vi "number1-state machine.vi"() -> ()   [LabVIEW 2014]
panel:
  out "Logined":bool
  in  "stop":bool
  out "array":bool[](array[boolean])
  in  "Button":T1
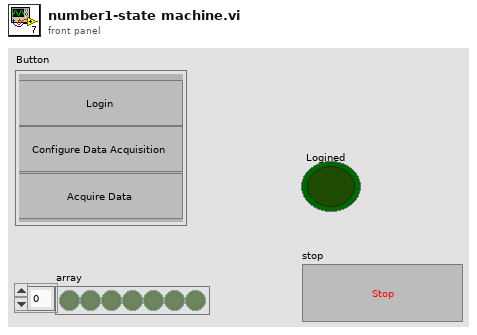
[diagram p1: front panel]
types:
  T1 = cluster{"OK Button":bool, "OK Button 2":bool, "OK Button 3":bool}
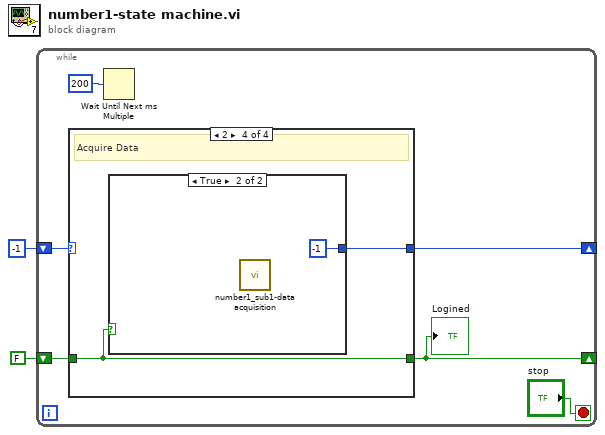
[diagram p0: block diagram]
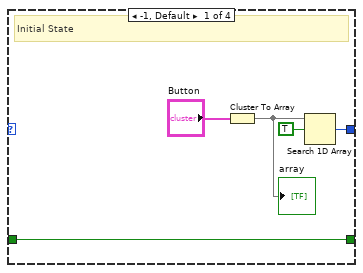
[diagram p2: hidden frame]
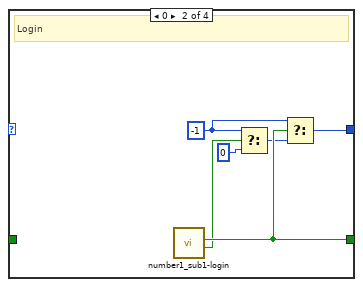
[diagram p3: hidden frame]
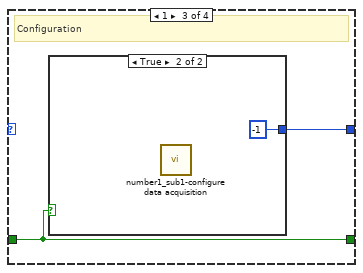
[diagram p4: hidden frame]
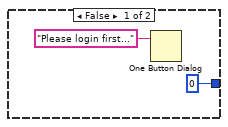
[diagram p5: hidden frame]
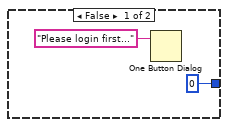
[diagram p6: hidden frame]
diagram:
  n1 = while {
    shift-right: [w7] -> _
    shift-left: -1 -> [w8]
    shift-right: [w6] -> _
    shift-left: FALSE -> [w5]
    stop <- "stop" stop-if-true
    n2 = case shown="2" w8 {
      tunnel: [w10 w18 w20 w25] -> w7
      tunnel: [w9 w19 w21 w26] -> w6
      tunnel: w5 -> [w9 _ w21 w26]
      frame -1, Default {
        # "Initial State"
        n3 = Cluster To Array(cluster="Button") -> (array=w12:bool[])
        "array" <- w12
        n4 = Search 1D Array(1D array=w12, element=TRUE) -> (index of element=w10:i32)  [unwired: 1 in]
      }
      frame 0 {
        w16 = -1
        # "Login"
        n5 = call "number1_sub1-login.vi"() -> ("UserCancelled"=w17:bool, "Correct"=w19:bool)  [unwired: 10 in]
        n6 = Select(t=w16, s=w17, f=0) -> (s? t:f=w14:i32)
        n7 = Select(t=w16, s=w19, f=w14) -> (s? t:f=w18:i32)
      }
      frame 1 {
        # "Configuration"
        n8 = case shown="True" w21 {
          tunnel: [0 -1] -> w20
          frame False {
            n9 = One Button Dialog(message="Please login first...") -> ()  [unwired: 1 in, 1 out]
          }
          frame True {
            n10 = call "number1_sub1-configure data acquisition.vi"() -> ()  [unwired: 8 in]
          }
        }
      }
      frame 2 {
        # "Acquire Data"
        n11 = case shown="True" w26 {
          tunnel: [0 -1 ("index of element")] -> w25
          frame False {
            n12 = One Button Dialog(message="Please login first...") -> ()  [unwired: 1 in, 1 out]
          }
          frame True {
            n13 = call "number1_sub1-data acquisition.vi"() -> ()  [unwired: 5 in, 1 out]
          }
        }
      }
    }
    "Logined" <- w6
    n14 = Wait Until Next ms Multiple(millisecond multiple=u32 200) -> ()  [unwired: 1 out]
  }
